vi "2 Ch Digital Output.vi"(2 "Packet":u64, 4 "2 Ch Digital Out":cluster{"DO0":refnum<k21>, "DO1":refnum<k21>}={"DO0"="Chassis1/Mod3/DO0", "DO1"="Chassis1/Mod3/DO1"}) -> ()   [LabVIEW 2009]
uses:
  <vilib>/eio/EIONode/EIONode.xnode
  <vilib>/rvi/eio/nirviEIOImplementation/nirviEIOImplementation.xnode
  <vilib>/rvi/eio/common/nirviEmuTemplateMethod_noerrors.vi
  <vilib>/rvi/eio/common/nirviEmuClasses.ctl
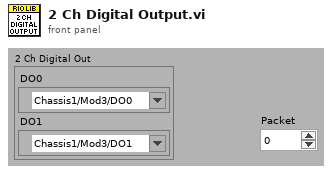
[diagram p1: front panel]
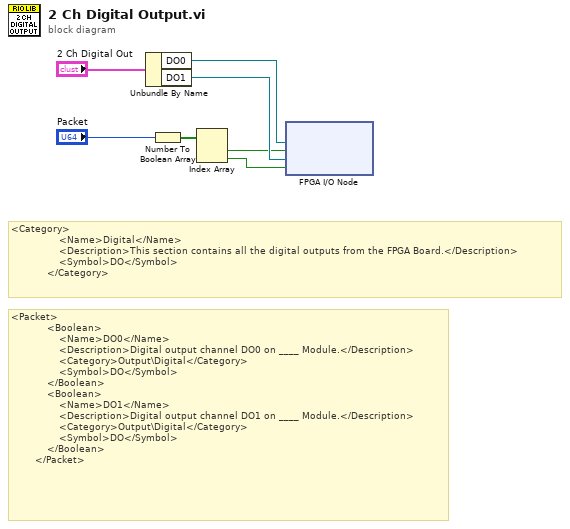
[diagram p0: block diagram]
diagram:
  # "<Category>\n                <Name>Digital</Name>\n                <Description>This section contains all the digital outputs from the FPGA Board.</Description>\n                <Symbol>DO</Symbol>\n            </Category>"
  # "<Packet>\n            <Boolean>\n                <Name>DO0</Name>\n                <Description>Digital output channel DO0 on ____ Module.</Description>\n                <Category>Output\\Digital</Category>\n                <Symbol>DO</Symbol>\n            </Boolean>\n            <Boolean>\n                <Name>DO1</Name>\n                <Description>Digital output channel DO1 on ____ Module.</Description>\n                <Category>Output\\Digital</Category>\n                <Symbol>DO</Symbol>\n            </Boolean>\n        </Packet>"
  n1 = Unbundle By Name("2 Ch Digital Out") -> ("DO0"=w6:refnum<k21>, "DO1"=w7:refnum<k21>)
  n2 = Number To Boolean Array(number="Packet") -> (Boolean array=w2:bool[])
  n3 = Index Array(array=w2) -> (element #1=w3:bool, element #2=w4:bool)  [unwired: 2 in]
  n4 = xnode "FPGA I/O Node"("I/O Item"=w3, "I/O Item"=w4, "FPGA I/O In"=w6, "FPGA I/O In"=w7) -> ()  [unwired: 2 out]
